vi "4_3_MNIST_Inference(FPGA)(RT).vi"() -> ()   [LabVIEW 2020]
doc: "This example demonstrates the usage of \"DeepLTK FPGA Addon\" for loading the model pretrained for handwritten digit recognition and running for inference on sbRIO-9609 by utilizing FPGA as an accelerator.\n\nMore Examples: https://github.com/ngenehub/deepltk_fpga_examples"
uses:
  <vilib>/Ngene/DeepLTK FPGA Addon/Toolkit/NNF_Host/Low_Level/NNF_Init/Controls/NNF_FPGA_Target_Info.ctl
  <vilib>/userDefined/High Color/nirio_resource_hc.ctl
  <vilib>/FPGAPlugInAG/Dynamic/niLvFpga_Download_Dynamic.vi
  <vilib>/FPGAPlugInAG/Dynamic/niLvFpga_Run_Dynamic.vi
  <vilib>/Ngene/DeepLTK FPGA Addon/Toolkit/NNF_Host/API/NNF_Set_Input/NNF_Set_Input(2D_I8).vi
  <vilib>/FPGAPlugInAG/Dynamic/niLvFpga_Close_Dynamic.vi
  <vilib>/rvi/interface/nirviMethod/nirviMethod.xnode
  <vilib>/rvi/interface/nirviCloseFPGA/nirviCloseFPGA.xnode
  <vilib>/Ngene/Deep Learning Toolkit/Toolkit/Deep_Learning_Toolkit_by_Ngene.lvlib
  <vilib>/Ngene/DeepLTK FPGA Addon/Toolkit/DeepLTK_FPGA_Addon.lvlib
  <vilib>/ptbypt/NI_PtbyPt.lvlib
panel:
  in  "FPGA Target":T1="RIO0" caption="RIO Device"
  out "Target Information":T2={"BRAM _Buff_1_Size"=52500, "BRAM _Buff_2_Size"=45937, "Version"=[8, 1, 1, 0], "# Cores"=8}
  in  "FPGA Bitfile":path=path "c:/DeepLTK_FPGA_Addon/NNF_sbRIO_9609_8Cores.lvbitx"
  in  "Scalers File Path":path=path "c:/DeepLTK_FPGA_Addon/models/MNIST_NNF_Converted/mnist_cnn/NNF_mnist_cnn_net_scalers_24_11_25__15_36_06.cfg"
  out "Lables":string[](array[string])=["0", "1", "2", "3", "4", "5", "6", "7", "8", "9"]
  in  "Configuration File Path":path=path "c:/DeepLTK_FPGA_Addon/models/MNIST_NNF_Converted/mnist_cnn/NNF_mnist_cnn_net_cfg_24_11_25__15_36_06.cfg"
  in  "Weight File Path":path=path "c:/DeepLTK_FPGA_Addon/models/MNIST_NNF_Converted/mnist_cnn/NNF_mnist_cnn_weights_24_11_25__15_36_06.bin"
  in  "Image (28x28px)":sgl[][](graph)=[[-1.0, -1.0, -1.0, -1.0, -1.0, -1.0, -1.0, -1.0, -1.0, -1.0, -1.0, -1.0, -1.0, -1.0, -1.0, -1.0, -1.0, -1.0, -1.0, -1.0, -1.0, -1.0, -1.0, -1.0, -1.0, -1.0, -1.0, -1.0], [-1.0, -1.0, -1.0, -1.0, -1.0, -1.0, -1.0, -1.0, -1.0, -1.0, -1.0, -1.0, -1.0, -1.0, -1.0, -1.0, -1.0, -1.0, -1.0, -1.0, -1.0, -1.0, -1.0, -1.0, -1.0, -1.0, -1.0, -1.0], [-1.0, -1.0, -1.0, -1.0, -1.0, -1.0, -1.0, -1.0, -1.0, -1.0, -1.0, -1.0, -1.0, -1.0, -1.0, -1.0, -1.0, -1.0, -1.0, -1.0, -1.0, -1.0, -1.0, -1.0, -1.0, -1.0, -1.0, -1.0], [-1.0, -1.0, -1.0, -1.0, -1.0, -1.0, -1.0, -1.0, -1.0, -1.0, -1.0, -1.0, -1.0, -1.0, -1.0, -1.0, -1.0, -1.0, -1.0, -1.0, -1.0, -1.0, -1.0, -1.0, -1.0, -1.0, -1.0, -1.0], [-1.0, -1.0, -1.0, -1.0, -1.0, -1.0, -1.0, -1.0, -0.7992126, 0.003937008, -0.6185039, -1.0, -1.0, -1.0, -1.0, -1.0, -1.0, -1.0, -1.0, -1.0, -1.0, -1.0, -1.0, -1.0, -1.0, -1.0, -1.0, -1.0], [-1.0, -1.0, -1.0, -1.0, -1.0, -1.0, -1.0, -1.0, 0.24488188, 1.007874, 0.5661417, -1.0, -1.0, -1.0, -1.0, -1.0, -1.0, -1.0, -1.0, -1.0, -1.0, -1.0, -1.0, -1.0, -1.0, -1.0, -1.0, -1.0], [-1.0, -1.0, -1.0, -1.0, -1.0, -1.0, -1.0, -1.0, 0.4055118, 1.007874, 0.42559054, -1.0, -1.0, -1.0, -1.0, -1.0, -1.0, -1.0, -1.0, -1.0, -1.0, -1.0, -1.0, -1.0, -1.0, -1.0, -1.0, -1.0], [-1.0, -1.0, -1.0, -1.0, -1.0, -1.0, -1.0, -1.0, 0.4055118, 1.007874, 0.4055118, -1.0, -1.0, -1.0, -1.0, -1.0, -1.0, -1.0, -1.0, -1.0, -1.0, -1.0, -1.0, -1.0, -1.0, -1.0, -1.0, -1.0], [-1.0, -1.0, -1.0, -1.0, -1.0, -1.0, -1.0, -1.0, 0.4055118, 1.007874, 0.4055118, -1.0, -1.0, -1.0, -1.0, -1.0, -1.0, -1.0, -1.0, -1.0, -1.0, -1.0, -1.0, -1.0, -1.0, -1.0, -1.0, -1.0], [-1.0, -1.0, -1.0, -1.0, -1.0, -1.0, -1.0, -1.0, 0.4055118, 1.007874, 0.4055118, -1.0, -1.0, -1.0, -1.0, -1.0, -1.0, -1.0, -1.0, -1.0, -1.0, -1.0, -1.0, -1.0, -1.0, -1.0, -1.0, -1.0], [-1.0, -1.0, -1.0, -1.0, -1.0, -1.0, -1.0, -1.0, 0.58622044, 1.007874, 0.32519686, -1.0, -1.0, -1.0, -1.0, -0.8393701, 0.78700787, 0.68661416, -0.91968507, -1.0, -1.0, -1.0, -1.0, -1.0, -1.0, -1.0, -1.0, -1.0], [-1.0, -1.0, -1.0, -1.0, -1.0, -1.0, -1.0, -1.0, 0.7468504, 1.007874, 0.16456693, -1.0, -1.0, -1.0, -1.0, -0.538189, 1.007874, 1.007874, -0.33740157, -1.0, -1.0, -1.0, -1.0, -1.0, -1.0, -1.0, -1.0, -1.0], [-1.0, -1.0, -1.0, -1.0, -1.0, -1.0, -1.0, -1.0, 0.9275591, 1.007874, -0.11653543, -1.0, -1.0, -1.0, -1.0, -0.9598425, 0.9275591, 1.007874, 0.28503937, -1.0, -1.0, -1.0, -1.0, -1.0, -1.0, -1.0, -1.0, -1.0], [-1.0, -1.0, -1.0, -1.0, -1.0, -1.0, -1.0, -0.87952757, 1.007874, 1.007874, -0.21692914, -1.0, -1.0, -1.0, -1.0, -1.0, 0.6062992, 1.007874, 0.82716537, -1.0, -1.0, -1.0, -1.0, -1.0, -1.0, -1.0, -1.0, -1.0], [-1.0, -1.0, -1.0, -1.0, -1.0, -1.0, -1.0, -0.7992126, 1.007874, 1.007874, -0.39763778, -1.0, -1.0, -1.0, -1.0, -1.0, 0.6062992, 1.007874, 1.007874, -0.91968507, -1.0, -1.0, -1.0, -1.0, -1.0, -1.0, -1.0, -1.0], [-1.0, -1.0, -1.0, -1.0, -1.0, -1.0, -1.0, -0.5984252, 1.007874, 1.007874, -0.4980315, -1.0, -1.0, -1.0, -1.0, -1.0, 0.70669293, 1.007874, 1.007874, -0.5582677, -1.0, -1.0, -1.0, -1.0, -1.0, -1.0, -1.0, -1.0], [-1.0, -1.0, -1.0, -1.0, -1.0, -1.0, -1.0, -0.5984252, 1.007874, 1.007874, 0.5259842, 0.4055118, 0.4055118, 0.4055118, 0.4055118, 0.48582676, 1.007874, 1.007874, 1.007874, -0.13661417, -1.0, -1.0, -1.0, -1.0, -1.0, -1.0, -1.0, -1.0], [-1.0, -1.0, -1.0, -1.0, -1.0, -1.0, -1.0, -0.8393701, 0.9476378, 1.007874, 1.007874, 1.007874, 1.007874, 1.007874, 1.007874, 1.007874, 1.007874, 1.007874, 1.007874, -0.07637795, -1.0, -1.0, -1.0, -1.0, -1.0, -1.0, -1.0, -1.0], [-1.0, -1.0, -1.0, -1.0, -1.0, -1.0, -1.0, -1.0, -0.2972441, 0.4055118, 0.4055118, 0.4055118, 0.4055118, 0.4055118, 0.4055118, 0.34527558, -0.036220472, 1.007874, 1.007874, -0.17677166, -1.0, -1.0, -1.0, -1.0, -1.0, -1.0, -1.0, -1.0], [-1.0, -1.0, -1.0, -1.0, -1.0, -1.0, -1.0, -1.0, -1.0, -1.0, -1.0, -1.0, -1.0, -1.0, -1.0, -1.0, -1.0, 0.8070866, 1.007874, 0.003937008, -1.0, -1.0, -1.0, -1.0, -1.0, -1.0, -1.0, -1.0], [-1.0, -1.0, -1.0, -1.0, -1.0, -1.0, -1.0, -1.0, -1.0, -1.0, -1.0, -1.0, -1.0, -1.0, -1.0, -1.0, -1.0, 0.8070866, 1.007874, 0.14448819, -1.0, -1.0, -1.0, -1.0, -1.0, -1.0, -1.0, -1.0], [-1.0, -1.0, -1.0, -1.0, -1.0, -1.0, -1.0, -1.0, -1.0, -1.0, -1.0, -1.0, -1.0, -1.0, -1.0, -1.0, -1.0, 0.72677165, 1.007874, 0.14448819, -1.0, -1.0, -1.0, -1.0, -1.0, -1.0, -1.0, -1.0], [-1.0, -1.0, -1.0, -1.0, -1.0, -1.0, -1.0, -1.0, -1.0, -1.0, -1.0, -1.0, -1.0, -1.0, -1.0, -1.0, -1.0, 0.6062992, 1.007874, 0.26496062, -1.0, -1.0, -1.0, -1.0, -1.0, -1.0, -1.0, -1.0], [-1.0, -1.0, -1.0, -1.0, -1.0, -1.0, -1.0, -1.0, -1.0, -1.0, -1.0, -1.0, -1.0, -1.0, -1.0, -1.0, -1.0, 0.6062992, 1.007874, 0.32519686, -1.0, -1.0, -1.0, -1.0, -1.0, -1.0, -1.0, -1.0], [-1.0, -1.0, -1.0, -1.0, -1.0, -1.0, -1.0, -1.0, -1.0, -1.0, -1.0, -1.0, -1.0, -1.0, -1.0, -1.0, -1.0, 0.6062992, 1.007874, 0.20472442, -1.0, -1.0, -1.0, -1.0, -1.0, -1.0, -1.0, -1.0], [-1.0, -1.0, -1.0, -1.0, -1.0, -1.0, -1.0, -1.0, -1.0, -1.0, -1.0, -1.0, -1.0, -1.0, -1.0, -1.0, -1.0, 0.6062992, 1.007874, 0.20472442, -1.0, -1.0, -1.0, -1.0, -1.0, -1.0, -1.0, -1.0], [-1.0, -1.0, -1.0, -1.0, -1.0, -1.0, -1.0, -1.0, -1.0, -1.0, -1.0, -1.0, -1.0, -1.0, -1.0, -1.0, -1.0, 0.08425197, 1.007874, -0.11653543, -1.0, -1.0, -1.0, -1.0, -1.0, -1.0, -1.0, -1.0], [-1.0, -1.0, -1.0, -1.0, -1.0, -1.0, -1.0, -1.0, -1.0, -1.0, -1.0, -1.0, -1.0, -1.0, -1.0, -1.0, -1.0, -1.0, -0.81929135, -1.0, -1.0, -1.0, -1.0, -1.0, -1.0, -1.0, -1.0, -1.0]]
  out "Test Speed (img/s)":dbl=1287.9832706427546 format="%#_3p"
  out "test time(s/img)":dbl=0.0007764076000000841 format="%#_3p"
  out "Predictions":sgl[](array[slide])=[2.587976e-06, 0.00010891199, 6.734085e-07, 1.5088008e-07, 0.9998122, 6.734085e-07, 1.5578851e-05, 2.1011872e-05, 1.970869e-09, 3.8222883e-05] scale=0.0..1.0
  in  "Stop":bool
  # "Overview: This example demonstrates the usage of \"DeepLTK FPGA Addon\" for loading the model pretrained for handwritten digit recognition and running for inference on sbRIO by utilizing FPGA as an accelerator.\nRequirements: \n•DeepLTK - Deep Learning Toolkit for LabVIEW (https://www.ngene.co/deep-learning-toolkit-for-labview)\n•DeepLTK FPGA Addon (https://www.ngene.co/deepltk-accelerator-for-fpga)\n•NI FPGA Module                       \nInstructions:\nThis example runs in parallel with \"1_Drawing_Interface.vi \", which is required to generate test image samples.\n1.\tCopy the target-compatible FPGA bitfile (from project or compiled) on the development machine\n2.\tCopy converted model on the development machine.\n3.\tSelect FPGA target at FPGA Target control.\n4.\tProvide path to compiled FPGA bitfile at FPGA Bitfile control.\n5.\tProvide paths to .cfg, .bin and scalers.cfg files generated during model conversion at Network Configuration File Path, Weight File Path and Scalers File Path controls.\n6.\tRun the VI.\n7.\tDraw a digit in \"4_1_MNIST_Drawing_Interface(CPU).vi\" and copy the data from \"Image (28x28px)\" indicator.\n8.\tIn this VI right-click on \"Image (28x28px)\" control and select \"Paste Data\".\n9.\tObserve the \"Predictions\" results and the inference speed/time.\nMore Examples: https://github.com/ngenehub/deepltk_fpga_examples"
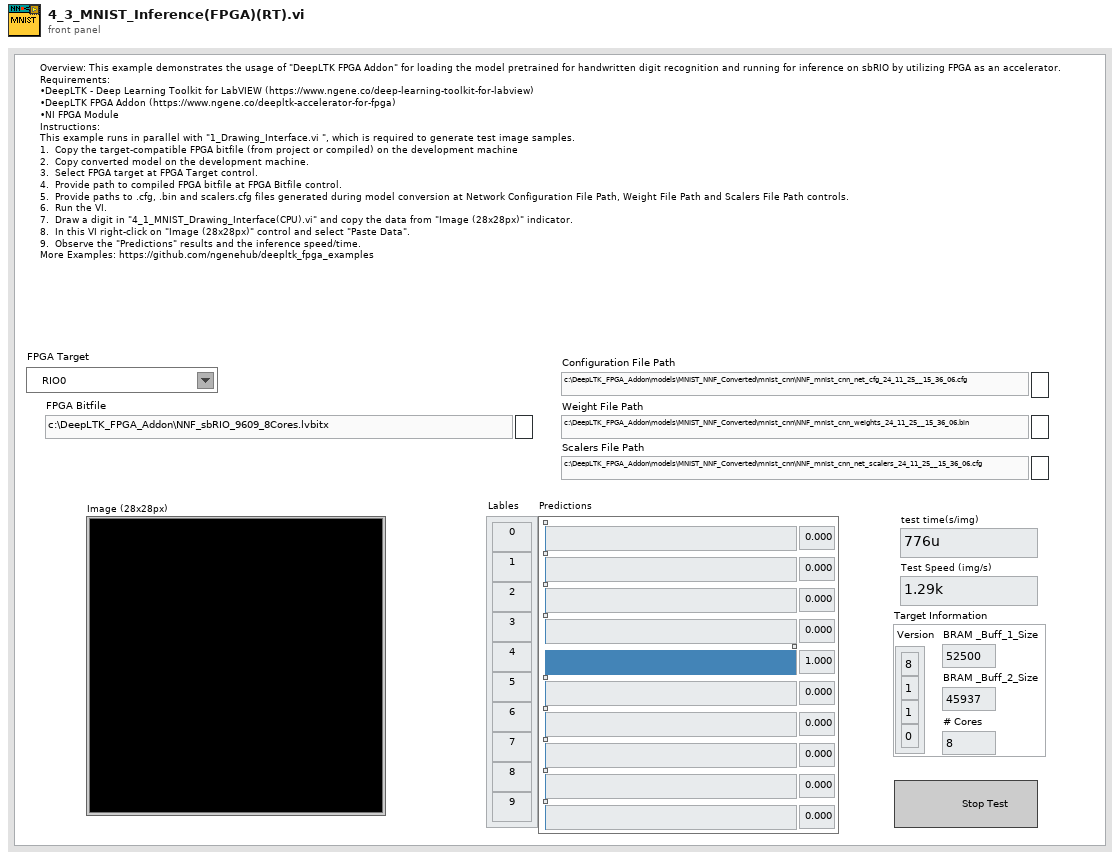
[diagram p1: front panel]
types:
  T1 = typedef "nirio_resource_hc.ctl" = tag
  T2 = typedef "DeepLTK_FPGA_Addon.lvlib/NNF_FPGA_Target_Info.ctl" = cluster{"BRAM _Buff_1_Size":u32, "BRAM _Buff_2_Size":u32, "Version":u8[], "# Cores":u32}
  T3 = typedef "DeepLTK_FPGA_Addon.lvlib/NNF.ctl" = cluster{"FPGA VI Ref ":refnum<k20>, "Subnets":T4[], "Dims_In":T6, "#Cores(enum)":T7, "NN_Ref":T8}
  T4 = typedef "DeepLTK_FPGA_Addon.lvlib/NNF_Subnet.ctl" = cluster{"Subnet Type":T5, "Subnet Data":variant, "Input Scaler":sgl, "Output Scaler":sgl}
  T5 = typedef "DeepLTK_FPGA_Addon.lvlib/NNF_Subnet_Type.ctl" = enum16{"CPU", "FPGA", "Split FPGA"}
  T6 = typedef "Deep_Learning_Toolkit_by_Ngene.lvlib/NN_Dims(C,H,W).ctl" = cluster{"C":i32, "H":i32, "W":i32}
  T7 = typedef "DeepLTK_FPGA_Addon.lvlib/NNF_No_Of_Cores.ctl" = enum16{"4CH", "8CH"}
  T8 = typedef "DeepLTK_FPGA_Addon.lvlib/NN_DVR.ctl" = refnum<data-value>
  T9 = typedef "Deep_Learning_Toolkit_by_Ngene.lvlib/NN_Layer.ctl" = cluster{"Name":string, "Layer_Data":variant, "Layer_Type":T10, "Dims_In":T6, "Layers_In":variant, "Dims_Out":T6, "Layers_Out":variant, "Metrics":T11, "GPU_Data":variant, "mBatch":i32, "NN_Device":T12, "NNg_hdls":T13, "Train?":bool, "Dimty":T14, "RecptField":T15}
  T10 = typedef "Deep_Learning_Toolkit_by_Ngene.lvlib/NN_Layer_Type.ctl" = enum16{"Input1D", "Input3D", "Conv1D", "Conv2D", "Conv2D_Adv", "MaxPool", "AvgPool", "UpSample", "DropOut3D", "ShortCut", "Concat", "SoftMax3D", "FC", "DropOut", "Softmax", "Flatten", "YOLO_v2", "YOLO_v4", "Activation", "BatchNormalization", "Unsupported"}
  T11 = typedef "Deep_Learning_Toolkit_by_Ngene.lvlib/NN_Layer_Metrics.ctl" = cluster{"Data":dbl, "Params":dbl, "Ops":dbl}
  T12 = typedef "Deep_Learning_Toolkit_by_Ngene.lvlib/NN_Device.ctl" = enum16{"CPU", "GPU"}
  T13 = typedef "Deep_Learning_Toolkit_by_Ngene.lvlib/nng_cuda_handles.ctl" = cluster{"cudnn":u64, "cublas":u64, "stream":u64, "curand":u64}
  T14 = typedef "Deep_Learning_Toolkit_by_Ngene.lvlib/NN_Layer_Dimty.ctl" = enum16{"1D", "3D"}
  T15 = typedef "Deep_Learning_Toolkit_by_Ngene.lvlib/NN_Layer_RF_State.ctl" = cluster{"Dims":T16, "J":T16}
  T16 = typedef "Deep_Learning_Toolkit_by_Ngene.lvlib/NN_Dims(V,H).ctl" = cluster{"V":i32, "H":i32}
  T17 = typedef "Deep_Learning_Toolkit_by_Ngene.lvlib/NN.ctl" = cluster{"Name":string, "No of Layers":i32, "mBatch":i32, "Layers":T18[], "Dimty":T19, "Dims_In":T6, "Dims_Out":T6, "Working_Dir":path, "Train?":bool, "Train_Params":T20, "LR_Update_Policy":T23, "Session Data":T25, "Ground_truth":T26, "NNg_hdls":T13, "NN_Device":T12, "GPU Id":i32, "Labels":string[], "Receptive Field":T16[], "Loss_Type":T27, "Loss_Cfg_Prms":variant, "NNG_WS":T28}
  T18 = typedef "Deep_Learning_Toolkit_by_Ngene.lvlib/NN_Layer_ref.ctl" = refnum<data-value>
  T19 = typedef "Deep_Learning_Toolkit_by_Ngene.lvlib/NN_In_Out_Dim-ty.ctl" = enum8{"In1D_Out1D", "In3D_Out1D", "In3D_Out3D", "In3D_OutBBox"}
  T20 = typedef "Deep_Learning_Toolkit_by_Ngene.lvlib/NN_Train_Params.ctl" = cluster{"Optimizer":T21, "Beta_1":sgl, "Beta_2":sgl, "Weight Decay(L1)":sgl, "Weight Decay(L2)":sgl, "Data_Sampling":T22}
  T21 = typedef "Deep_Learning_Toolkit_by_Ngene.lvlib/NN_Train_Optimizer.ctl" = enum16{"SGD", "Adam", "Adagrad", "Adadelta", "RMSProp", "Nesterov"}
  T22 = typedef "Deep_Learning_Toolkit_by_Ngene.lvlib/NN_Train_Data_Sampling.ctl" = enum16{"Random", "Sequential"}
  T23 = typedef "Deep_Learning_Toolkit_by_Ngene.lvlib/NN_LR_Policy_Cfg.ctl" = cluster{"Policy_Type":T24, "LR0":dbl, "k":sgl, "WarmUp_Policy":enum16{"Step", "Ramp"}, "WarmUp_Iter":i32, "WarmUp_Ratio":sgl}
  T24 = typedef "Deep_Learning_Toolkit_by_Ngene.lvlib/NN_LR_Policy_Type.ctl" = enum16{"Manual", "Step", "Exp", "1/t"}
  T25 = typedef "Deep_Learning_Toolkit_by_Ngene.lvlib/NN_Train_Session_Data.ctl" = cluster{"Epochs":sgl, "Tot_Iter":i32, "LR":sgl, "LR_iter":i32}
  T26 = typedef "Deep_Learning_Toolkit_by_Ngene.lvlib/NN_Ground_truth.ctl" = cluster{"Y":variant}
  T27 = typedef "Deep_Learning_Toolkit_by_Ngene.lvlib/NN_Loss_Type.ctl" = enum16{"None", "MSE", "CrossEntropy", "YOLO_v2", "YOLO_v4"}
  T28 = typedef "Deep_Learning_Toolkit_by_Ngene.lvlib/NNG_WS.ctl" = cluster{"NNG_WS_Mem":T29, "Max_WS_Size":i64}
  T29 = typedef "Deep_Learning_Toolkit_by_Ngene.lvlib/NNg_WS_Mem_DVR.ctl" = refnum<data-value>
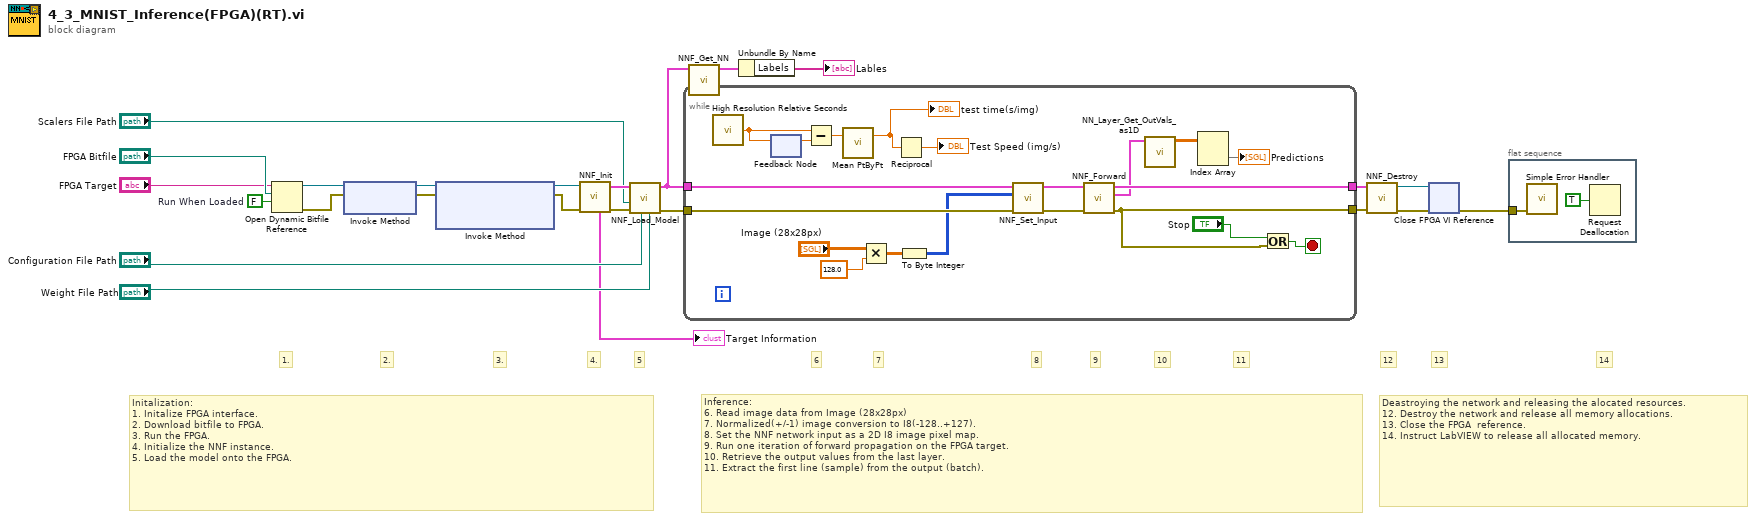
[diagram p0: block diagram]
diagram:
  w15 = FALSE  # Run When Loaded
  # "Deastroying the network and releasing the alocated resources. \n12. Destroy the network and release all memory allocations.\n13. Close the FPGA  reference.\n14. Instruct LabVIEW to release all allocated memory."
  # "14"
  # "13"
  # "12"
  # "11"
  # "10"
  # "9"
  # "8"
  # "7"
  # "6"
  # "5"
  # "4."
  # "Initalization:\n1. Initalize FPGA interface.\n2. Download bitfile to FPGA.\n3. Run the FPGA.\n4. Initialize the NNF instance.\n5. Load the model onto the FPGA."
  # "3."
  # "2."
  # "1."
  # "Inference:\n6. Read image data from Image (28x28px)\n7. Normalized(+/-1) image conversion to I8(-128..+127).\n8. Set the NNF network input as a 2D I8 image pixel map.\n9. Run one iteration of forward propagation on the FPGA target.\n10. Retrieve the output values from the last layer.\n11. Extract the first line (sample) from the output (batch)."
  n1 = Open Dynamic Bitfile Reference(0:"FPGA Target", 1:"FPGA Bitfile", 2:w15) -> (5:w17:refnum<k20>, 8:w13:errorcluster)  [unwired: 2 in]
  n2 = xnode "Invoke Method"("FPGA VI Reference In"=w17, "error in"=w13) -> ("FPGA VI Reference Out"=w14:refnum<k20>, "error out"=w11:errorcluster)
  n3 = xnode "Invoke Method"("FPGA VI Reference In"=w14, "error in"=w11) -> ("FPGA VI Reference Out"=w12:refnum<k20>, "error out"=w10:errorcluster)  [unwired: 1 in]
  n4 = call <vilib>:"NNF_Init.vi"("error in"=w10, "FPGA Interface"=w12) -> ("error out"=w23:errorcluster, "NNF out"=w16:T3, "Target Information"=→"Target Information":T2)  [unwired: 7 in]
  n5 = call <vilib>:"NNF_Load_Model.vi"("Weight File Path"="Weight File Path", "Network CFG File Path"="Configuration File Path", "Error in"=w23, "Scalers"="Scalers File Path", "NNF in"=w16) -> ("error Out"=w24:errorcluster, "NNF out"=w3:T3)  [unwired: 5 in]
  n6 = while {
    tunnel: w3 -> [w44]
    tunnel: w24 -> [w43]
    tunnel: [w40] -> w22
    tunnel: [w39] -> w21
    stop <- w38 stop-if-true
    n7 = call <vilib>:"High Resolution Relative Seconds.vi"() -> ("relative seconds"=w42:dbl)
    n8 = feedback #1() -> (w41:dbl)  [unwired: 1 in]
    n9 = feedback-in #1(w42) -> ()
    n10 = Subtract(x=w42, y=w41) -> (x-y=w28:dbl)
    n11 = call <vilib>:"Mean PtByPt.vi"("x"=w28) -> ("mean"=w26:dbl)  [unwired: 3 in, 1 out]
    "test time(s/img)" <- w26
    n12 = Multiply(x="Image (28x28px)", y=sgl 128.0 ("x")) -> (x*y=w33:sgl[][])
    n13 = Reciprocal(x=w26) -> (1/x=→"Test Speed (img/s)":dbl)
    n14 = To Byte Integer(number=w33) -> (8bit integer=w31:i8[][])
    n15 = call-poly <vilib>:"NNF_Set_Input.vi"("error in"=w43, "Data_in(2D_I8)"=w31, "NNF In"=w44) -> ("error out"=w34:errorcluster, "NNF out"=w35:T3)  [unwired: 7 in]
    n16 = call <vilib>:"NNF_Forward.vi"("error in"=w34, "NNF in"=w35) -> ("error out"=w39:errorcluster, "Last_Layer"=w37:T9, "NNF out"=w40:T3)  [unwired: 7 in]
    n17 = call <vilib>:"NN_Layer_Get_OutVals_as1D.vi"("Layer"=w37) -> ("Out(as1D)"=w36:sgl[][])  [unwired: 9 in, 1 out]
    n18 = Index Array(array=w36) -> (element=→"Predictions":sgl[])  [unwired: 2 in]
    n19 = Or(x="Stop", y=w39) -> (x .or. y?=w38:bool)
  }
  n20 = call "NNF_Get_NN.vi"("NNF in"=w3) -> ("NN out"=w2:T17)  [unwired: 10 in]
  n21 = Unbundle By Name(w2) -> ("Labels"=→"Lables":string[])
  n22 = call <vilib>:"NNF_Destroy.vi"("error in"=w21, "NNF in"=w22) -> ("error out"=w20:errorcluster, "FPGA VI Ref"=w18:refnum<k20>)  [unwired: 8 in]
  n23 = xnode "Close FPGA VI Reference"("FPGA VI Reference In"=w18, "error in"=w20) -> ("error out"=w19:errorcluster)
  n24 = flat-sequence {
    tunnel: w19 -> [w46]
    frame #0 {
      n25 = call <vilib>:"Simple Error Handler.vi"("error in (no error)"=w46) -> ()  [unwired: 4 in, 5 out]
      n26 = Request Deallocation(TRUE ("flag")) -> ()
    }
  }
